vi "FTP.vi"() -> ()   [LabVIEW 2019]
uses:
  <vilib>/WebDAVClient/Simple Put File.vi
  <vilib>/WebDAVClient/NI_WebDAV.lvlib
  <vilib>/WebDAVClient/Advanced/Get File.vi
  <vilib>/WebDAVClient/Advanced/Multi Event/Asynchronous Get File.vi
  <vilib>/WebDAVClient/Simple Get File.vi
panel:
  out "error out 5":errorcluster
  out "error out 4":errorcluster
  out "error out 3":errorcluster
  out "local file path out 2":path
  out "string":string
  out "local file path out":path
  out "error out 2":errorcluster
  out "error out":errorcluster
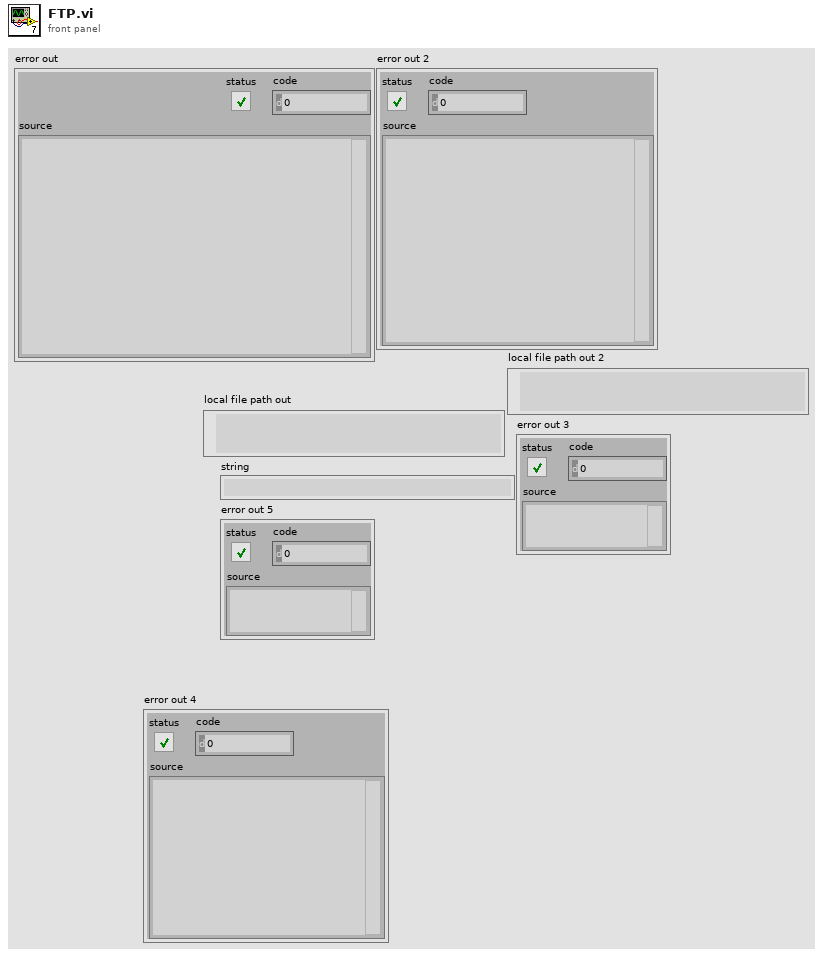
[diagram p1: front panel]
types:
  T1 = typedef "NI_WebDAV.lvlib/Asynchronous Session Handle.ctl" = refnum<k1>
  T2 = typedef "NI_WebDAV.lvlib/SessionHandle.ctl" = refnum<k1>
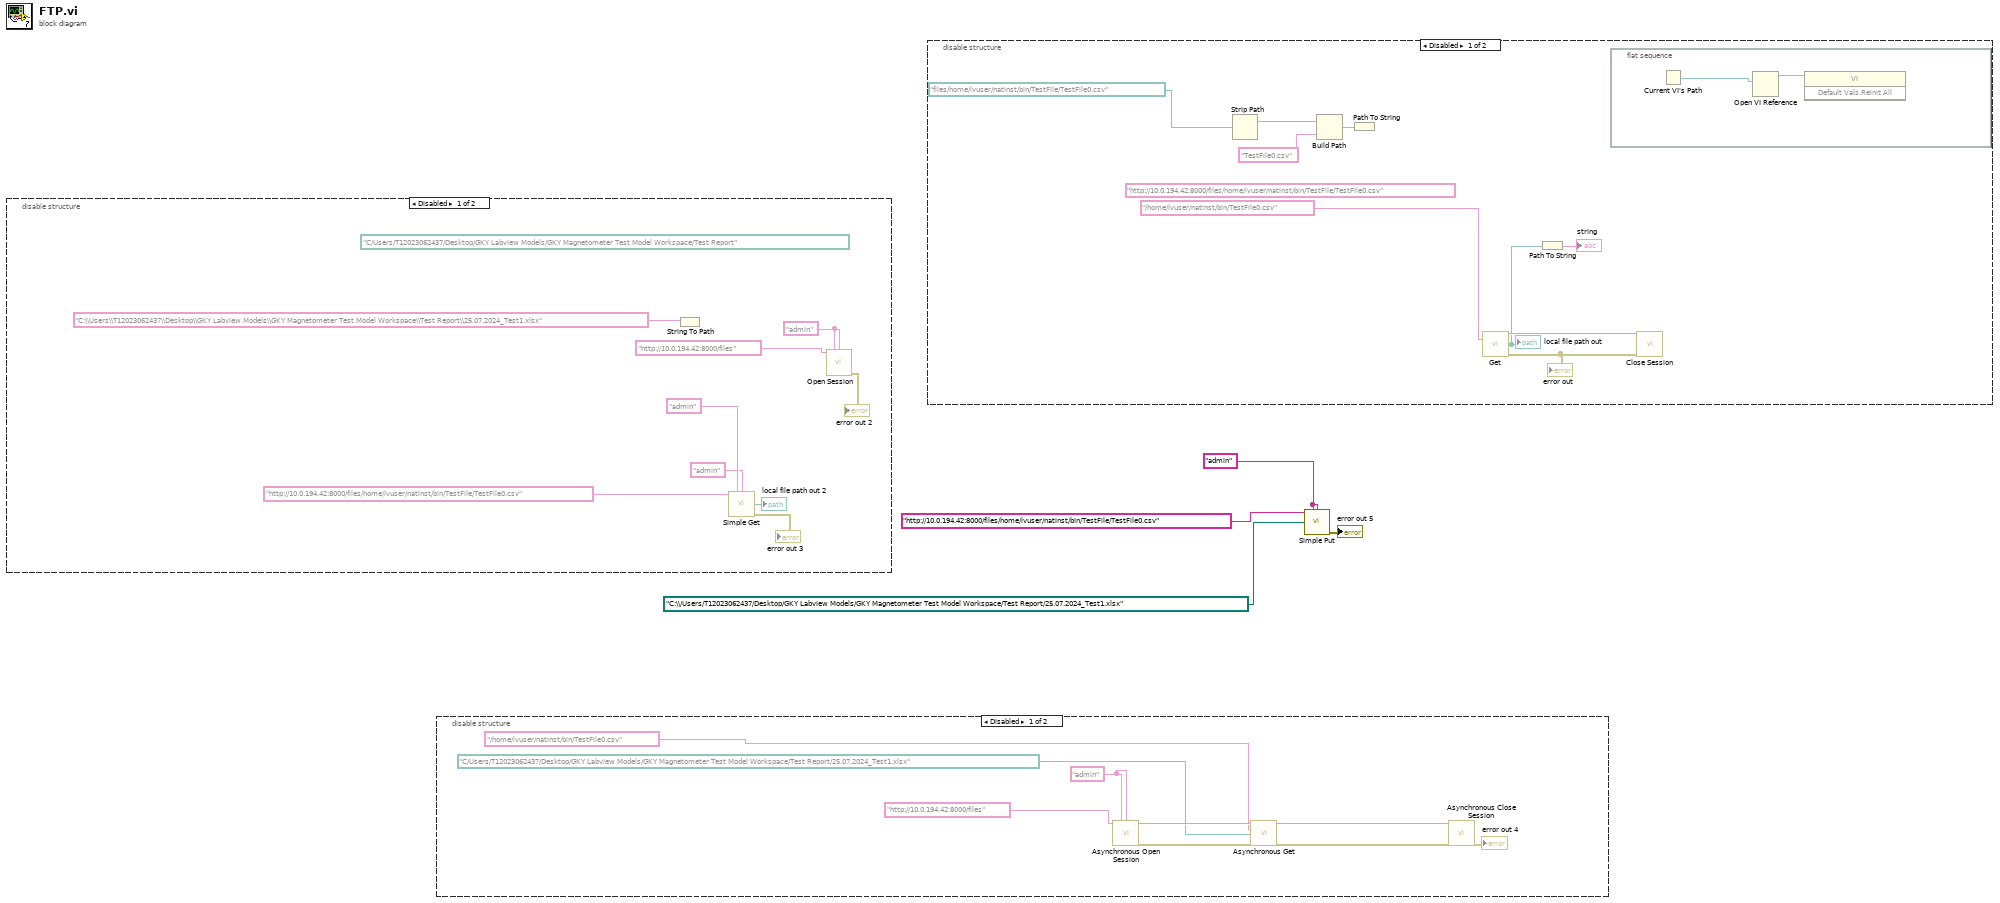
[diagram p0: block diagram]
diagram:
  w2 = "admin" ("password")
  n1 = disable-structure shown="Disabled" {
    frame Disabled {
      w10 = "admin" ("username")
      (unwired) path "C:/Users/T12023062437/Desktop/GKY Labview Models/GKY Magnetometer Test Model Workspace/Test Report" ("path")
      n2 = String To Path(string="C:\\Users\\T12023062437\\Desktop\\GKY Labview Models\\GKY Magnetometer Test Model Workspace\\Test Report\\25.07.2024_Test1.xlsx") -> ()  [unwired: 1 out]
      n3 = call-poly <vilib>:"Simple Get.vi"("remote file uri"="http://10.0.194.42:8000/files/home/lvuser/natinst/bin/TestFile/TestFile0.csv", "username"="admin", "password"="admin") -> ("local file path out"=→"local file path out 2":path, "error out"=→"error out 3":errorcluster)  [unwired: 11 in]
      n4 = call <vilib>:"Open Session.vi"("host uri prefix"="http://10.0.194.42:8000/files", "username"=w10, "password"=w10) -> ("error out"=→"error out 2":errorcluster)  [unwired: 11 in, 1 out]
    }
    frame Enabled {
    }
  }
  n5 = disable-structure shown="Disabled" {
    frame Disabled {
      w14 = "admin" ("username")
      n6 = call <vilib>:"Asynchronous Open Session.vi"("host uri prefix"="http://10.0.194.42:8000/files", "username"=w14, "password"=w14) -> ("session handle out"=w22:T1, "error out"=w21:errorcluster)  [unwired: 10 in, 1 out]
      n7 = call-poly <vilib>:"Asynchronous Get.vi"("session handle"=w22, "relative uri"="/home/lvuser/natinst/bin/TestFile0.csv", "local file path"=path "C:/Users/T12023062437/Desktop/GKY Labview Models/GKY Magnetometer Test Model Workspace/Test Report/25.07.2024_Test1.xlsx" ("path"), "error in (no error)"=w21) -> ("session handle out"=w20:T1, "error out"=w19:errorcluster)  [unwired: 8 in, 2 out]
      n8 = call <vilib>:"Asynchronous Close Session.vi"("session handle"=w20, "error in (no error)"=w19) -> ("error out"=→"error out 4":errorcluster)  [unwired: 13 in]
    }
    frame Enabled {
    }
  }
  n9 = disable-structure shown="Disabled" {
    frame Disabled {
      (unwired) "http://10.0.194.42:8000/files/home/lvuser/natinst/bin/TestFile/TestFile0.csv"
      n10 = Strip Path(path=path "/files/home/lvuser/natinst/bin/TestFile/TestFile0.csv") -> (stripped path=w29:path)  [unwired: 1 out]
      n11 = Build Path(base path=w29, name or relative path="TestFile0.csv") -> (appended path=w26:path)
      n12 = Path To String(path=w26) -> ()  [unwired: 1 out]
      n13 = call-poly <vilib>:"Get.vi"("relative uri"="/home/lvuser/natinst/bin/TestFile0.csv") -> ("session handle out"=w31:T2, "local file path out"=w24:path, "error out"=w30:errorcluster)  [unwired: 12 in]
      "error out" <- w30
      "local file path out" <- w24
      n14 = Path To String(path=w24) -> (string=→"string":string)
      n15 = flat-sequence {
        frame #0 {
          n16 = Current VI's Path() -> (path=w33:path)
          n17 = Open VI Reference(vi path=w33) -> (vi reference=w32:refnum<vi>)  [unwired: 5 in, 1 out]
          n18 = invoke class="VI" method="Default Vals.Reinit All"(reference=w32) -> ()  [unwired: 2 in, 3 out]
        }
      }
      n19 = call <vilib>:"Close Session.vi"("session handle"=w31, "error in (no error)"=w30) -> ()  [unwired: 13 in, 1 out]
    }
    frame Enabled {
    }
  }
  n20 = call-poly <vilib>:"Simple Put.vi"("file uri"="http://10.0.194.42:8000/files/home/lvuser/natinst/bin/TestFile/TestFile0.csv" ("remote file uri"), "username"=w2, "password"=w2, "local file path"=path "C:\\/Users/T12023062437/Desktop/GKY Labview Models/GKY Magnetometer Test Model Workspace/Test Report/25.07.2024_Test1.xlsx" ("path")) -> ("error out"=→"error out 5":errorcluster)  [unwired: 10 in, 1 out]
